vi "Method.vi"(4 "Value":refnum<class "Abs_U8 Integer.lvclass">) -> (1 "Result":refnum<class "Abs_Boolean.lvclass">)   [LabVIEW 2021, in "Greater Equal 0_U8.lvclass"]
uses:
  Greater Equal 0_U8.lvclass
  Abs_Types/U8 Integer/Abs_U8 Integer.lvclass
  Abs_Types/Boolean/Abs_Boolean.lvclass
  C:/TSA/LV_Abstract/Source/Functions/Support/Compare/One Term/U8/AbsComp_One Term_U8.lvclass
  C:/Program Files (x86)/National Instruments/LabVIEW 2021/vi.lib/TSA/Abstract Data Classes/Abs_Types/Boolean/Abs_Boolean.lvclass
  Support/Compare/One Term/U8/AbsComp_One Term_U8.lvclass/AbsComp_One Term_U8.ctl
  Support/Compare/One Term/U8/Properties/Write Numeric A.vi
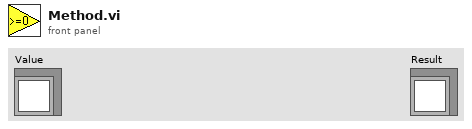
[diagram p1: front panel]
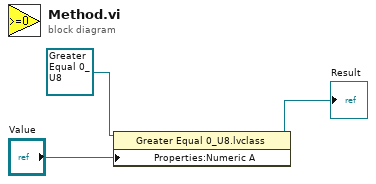
[diagram p0: block diagram]
diagram:
  n1 = property class="Greater Equal 0_U8.lvclass"(reference=refnum<class "Greater Equal 0_U8.lvclass"> refnum ("Greater 0_U64.lvclass"), "Properties:Numeric A"="Value") -> (reference out=→"Result":refnum<class "Greater Equal 0_U8.lvclass">)  [unwired: 1 in, 1 out]
